vi "Find Class by Name.vi"(8 "error in (no error)":errorcluster, 10 "Name":string, 11 "Installed Instruments":refnum<class "Instrument.lvclass">[](array[class])) -> (0 "error out":errorcluster, 3 "Instrument out":refnum<class "Instrument.lvclass">)   [LabVIEW 2019, in "Control Experiment.lvclass"]
uses:
  Control Experiment.lvclass
  <userlib>/LevyLab/Instrument Framework/Instrument/Instrument.lvclass
panel:
  out "Found?":bool[](array[boolean])
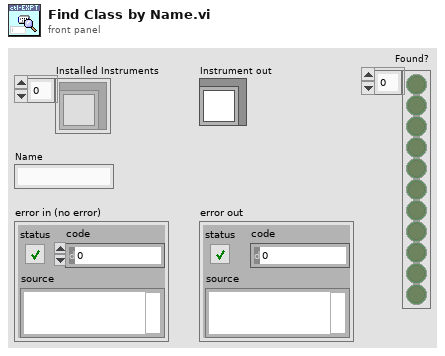
[diagram p1: front panel]
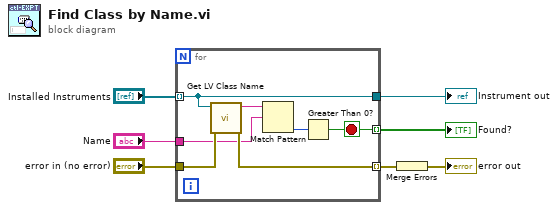
[diagram p0: block diagram]
diagram:
  n1 = for {
    tunnel: "Installed Instruments" -> [w13] mode=indexing
    tunnel: "Name" -> [w8]
    tunnel: [w13] -> w3
    tunnel: "error in (no error)" -> [w9]
    tunnel: [w12] -> w6 mode=indexing
    tunnel: [w10] -> w1 mode=indexing
    stop <- w10 stop-if-true
    n2 = call <vilib>:"Get LV Class Name.vi"("error in (no error)"=w9, "object"=w13) -> ("error out"=w12:errorcluster, "class name"=w11:string)  [unwired: 8 in]
    n3 = Match Pattern(string=w11, regular expression=w8) -> (offset past match=w14:i32)  [unwired: 1 in, 3 out]
    n4 = Greater Than 0?(x=w14) -> (x > 0?=w10:bool)
  }
  "Instrument out" <- w3
  "Found?" <- w1
  n5 = Merge Errors(w6) -> (→"error out":errorcluster)
